vi "Temp Control Test Program.vi"() -> ()   [LabVIEW 2022 SP3]
uses:
  Temp Control Parameters.ctl
  Temp Control.lvclass
  Lakeshore 325/Lakeshore 325.lvclass
  C:/Development/rimas/RIMAS/Temp Control/Temp Control/Temp Control.lvclass
  Lakeshore 331/Lakeshore 331.lvclass
  Lakeshore 218/Lakeshore 218.lvclass
  Lakeshore 336/Lakeshore 336.lvclass
panel:
  in  "Control Parameters":T1 {"Default Range" items=["Off", "Low (0.5W)", "Med (5W)", "High (50W)"]; "Heater Range" items=["Off", "Low (0.5W)", "Med (5W)", "High (50W)"]; "Manual Power (%)" format="%.3f"; "Mode" items=["Manual PID"=1, "Zone"=2, "Open Loop"=3, "AutoTune PID"=4, "AutoTune PI"=5, "AutoTune P"=6]}
  in  "Set Parameters":bool
  in  "Configure":bool
  in  "Set":bool
  in  "Addr":refnum<visa-resource-name>
  out "error out":errorcluster
  out "Data":dbl[](array[numeric])
  out "Channel Names":string[](array[string])=["Telescope RA", "Telescope DEC", "Telescope Moving?", "Telescope Status"]
  in  "LakeShore Model":T2(ring)
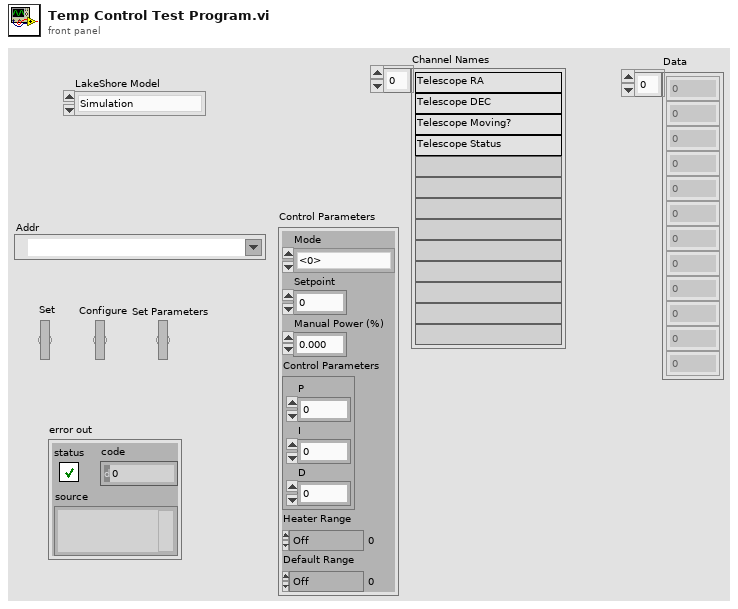
[diagram p1: front panel]
types:
  T1 = typedef "Temp Control.lvclass/Temp Control Parameters.ctl" = cluster{"Mode":u16, "Setpoint":dbl, "Manual Power (%)":dbl, "Control Parameters":cluster{"P":dbl, "I":dbl, "D":u16}, "Heater Range":u16, "Default Range":u16}
  T2 = enum16{"Simulation", "LakeShore 325", "LakeShore 331", "LakeShore 218", "LakeShore 336"}
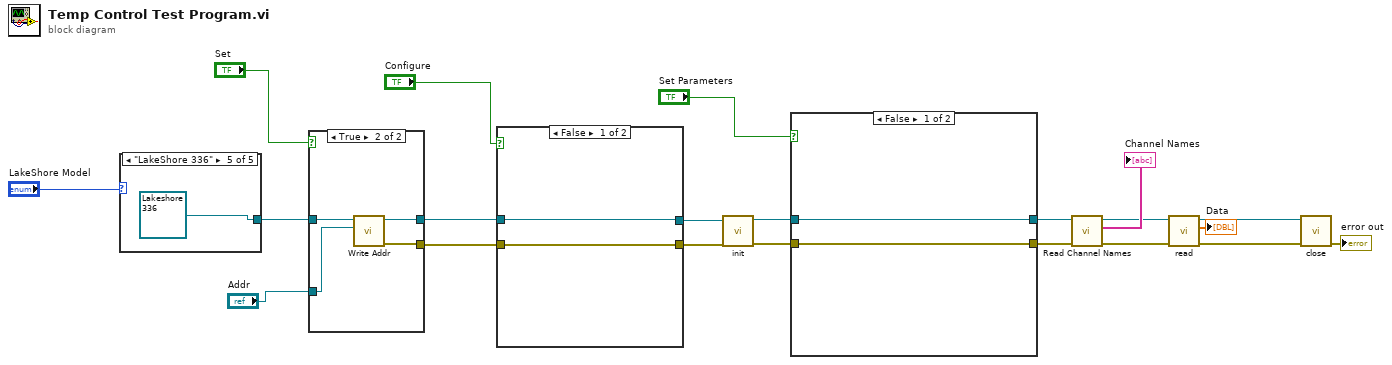
[diagram p0: block diagram]
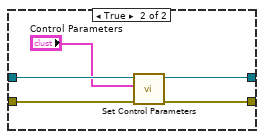
[diagram p2: hidden frame]
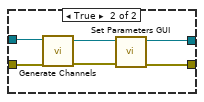
[diagram p3: hidden frame]
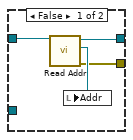
[diagram p4: hidden frame]
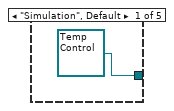
[diagram p5: hidden frame]
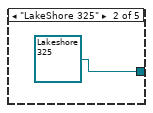
[diagram p6: hidden frame]
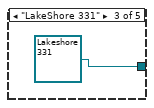
[diagram p7: hidden frame]
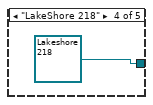
[diagram p8: hidden frame]
diagram:
  n1 = case shown="\"LakeShore 336\"" "LakeShore Model" {
    tunnel: [refnum<class "Temp Control.lvclass"> refnum ("Temp Control.lvclass") refnum<class "Lakeshore 325.lvclass"> refnum ("Lakeshore 325.lvclass") refnum<class "Lakeshore 331.lvclass"> refnum ("Lakeshore 331.lvclass") refnum<class "Lakeshore 218.lvclass"> refnum ("Lakeshore 218.lvclass") refnum<class "Lakeshore 336.lvclass"> refnum ("Lakeshore 336.lvclass")] -> w12
    frame "Simulation", Default {
    }
    frame "LakeShore 325" {
    }
    frame "LakeShore 331" {
    }
    frame "LakeShore 218" {
    }
    frame "LakeShore 336" {
    }
  }
  n2 = case shown="True" "Set" {
    tunnel: w12 -> [w30 w34]
    tunnel: [w29 w33] -> w9
    tunnel: "Addr" -> [_ w32]
    tunnel: [w27 w31] -> w8
    frame False {
      n3 = call-dynamic "Read Addr.vi"("Temp Control in"=w30) -> ("error out"=w27:errorcluster, "Addr"=w28:refnum<visa-resource-name>, "Temp Control out"=w29:refnum<class "Temp Control.lvclass">)  [unwired: 8 in]
      n4 = local write "Addr"(w28) -> ()
    }
    frame True {
      n5 = call-dynamic "Write Addr.vi"("Addr"=w32, "Temp Control in"=w34) -> ("error out"=w31:errorcluster, "Temp Control out"=w33:refnum<class "Temp Control.lvclass">)  [unwired: 8 in]
    }
  }
  n6 = case shown="False" "Configure" {
    tunnel: w9 -> [w36 w37]
    tunnel: w8 -> [w35 w40]
    tunnel: [w36 w42] -> w7
    tunnel: [w35 w41] -> w6
    frame False {
    }
    frame True {
      n7 = call-dynamic "Generate Channels.vi"("error in (no error)"=w40, "Temp Control in"=w37) -> ("error out"=w39:errorcluster, "Temp Control out"=w38:refnum<class "Temp Control.lvclass">)  [unwired: 6 in, 2 out]
      n8 = call-dynamic "Set Parameters GUI.vi"("error in (no error)"=w39, "Temp Control in"=w38) -> ("error out"=w41:errorcluster, "Temp Control out"=w42:refnum<class "Temp Control.lvclass">)  [unwired: 8 in]
    }
  }
  n9 = call-dynamic "init.vi"("error in (no error)"=w6, "Temp Control in"=w7) -> ("error out"=w4:errorcluster, "Temp Control out"=w3:refnum<class "Temp Control.lvclass">)  [unwired: 7 in, 1 out]
  n10 = case shown="False" "Set Parameters" {
    tunnel: w4 -> [w43 w49]
    tunnel: w3 -> [w44 w48]
    tunnel: [w44 w47] -> w2
    tunnel: [w43 w46] -> w1
    frame False {
    }
    frame True {
      n11 = call-dynamic "Set Control Parameters.vi"("error in (no error)"=w49, "Control Parameters"="Control Parameters", "Temp Control in"=w48) -> ("error out"=w46:errorcluster, "Temp Control out"=w47:refnum<class "Temp Control.lvclass">)  [unwired: 7 in]
    }
  }
  n12 = call-dynamic "Read Channel Names.vi"("error in (no error)"=w1, "Temp Control in"=w2) -> ("error out"=w17:errorcluster, "Channel Names"=→"Channel Names":string[], "Temp Control out"=w19:refnum<class "Temp Control.lvclass">)  [unwired: 7 in]
  n13 = call-dynamic "read.vi"("error in (no error)"=w17, "Temp Control in"=w19) -> ("error out"=w16:errorcluster, "Data"=→"Data":dbl[], "Temp Control out"=w18:refnum<class "Temp Control.lvclass">)  [unwired: 7 in]
  n14 = call-dynamic "close.vi"("error in (no error)"=w16, "Temp Control in"=w18) -> ("error out"=→"error out":errorcluster)  [unwired: 8 in, 1 out]
